vi "GetInitialBoard.vi"(8 "error in (no error)":errorcluster, 11 "GameRecorder in":refnum<class "GameRecorder.lvclass">) -> (0 "error out":errorcluster, 2 "TronviewGame.lvlib:Board":refnum<class "Board.lvclass">, 3 "GameRecorder out":refnum<class "GameRecorder.lvclass">)   [LabVIEW 2015, in "TronviewGame.lvlib" / "GameRecorder.lvclass"]
uses:
  GameRecorder.lvclass
  Board/Board.lvclass
  GameRecorder.lvclass/GameRecorder.ctl
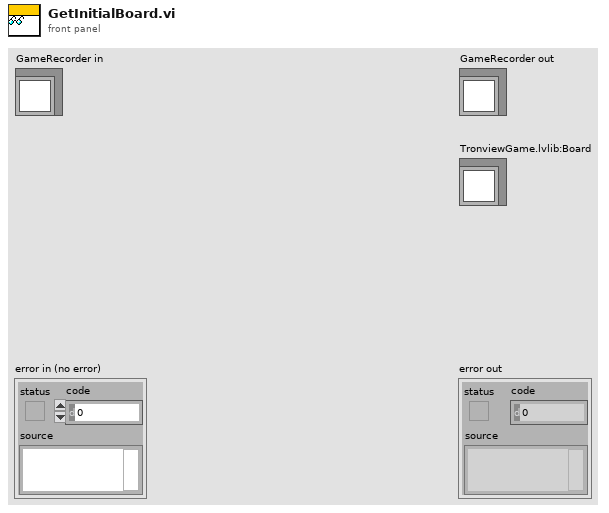
[diagram p1: front panel]
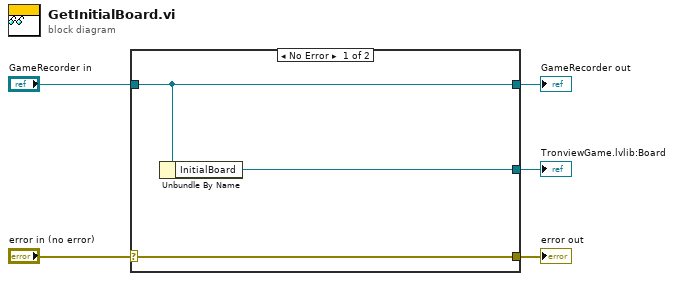
[diagram p0: block diagram]
diagram:
  n1 = case shown="No Error" "error in (no error)" {
    selector: "error in (no error)" -> [w8 w9]
    tunnel: [w8 w9] -> w4
    tunnel: [w7 w10] -> w2
    tunnel: "GameRecorder in" -> [w7 w10]
    tunnel: [w6 _] -> w1
    frame No Error {
      n2 = Unbundle By Name(w7) -> ("InitialBoard"=w6:refnum<class "Board.lvclass">)
    }
    frame Error {
    }
  }
  "error out" <- w4
  "GameRecorder out" <- w2
  "TronviewGame.lvlib:Board" <- w1
